vi "configure.vi"(8 "error in (no error)":errorcluster, 11 "SweepDL090926Automation in":refnum<class "SweepDL090926Automation.lvclass">) -> (0 "error out":errorcluster, 3 "SweepDL090926Automation out":refnum<class "SweepDL090926Automation.lvclass">)   [LabVIEW 2010, in "SweepDL090926Automation.lvclass"]
doc: "The dynamic dispatch version of this VI loads and displays the configuration file associated with the plug-in object. The user modify and save the configuration data."
uses:
  SweepDL090926Automation.lvclass
  ImagingMode/GenericImagingMode/GenericImagingMode/GenericImagingMode.lvclass
  SweepDL090926Automation.lvclass/SweepDL090926Automation.ctl
  common/classes/GenericComponent/GenericComponent/GenericComponent.lvclass
panel:
  in  "cancel button":bool
  in  "save button":bool
  in  "edit sequence button":bool
  # "Configure SweepDL090926Automation"
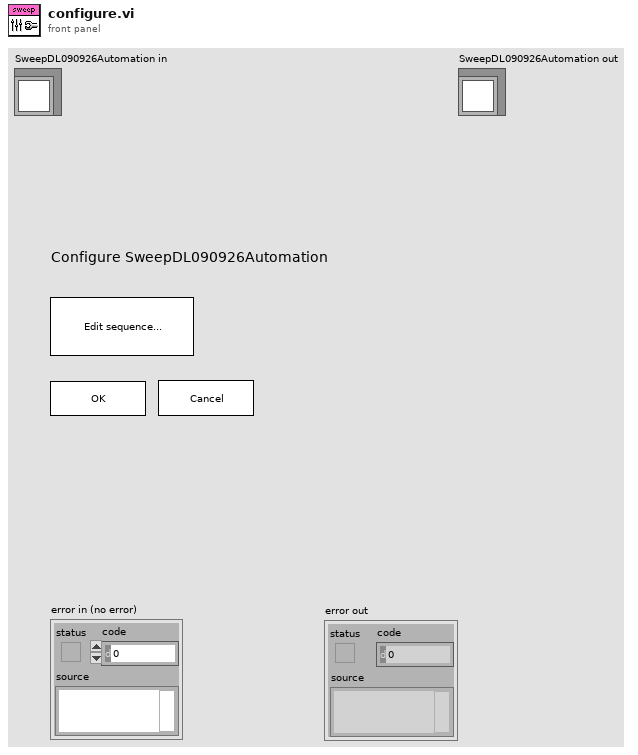
[diagram p1: front panel]
types:
  T1 = typedef "plugin_specification.ctl" = cluster{"class path":string, "configuration":string, "label":string, "settings name":string}
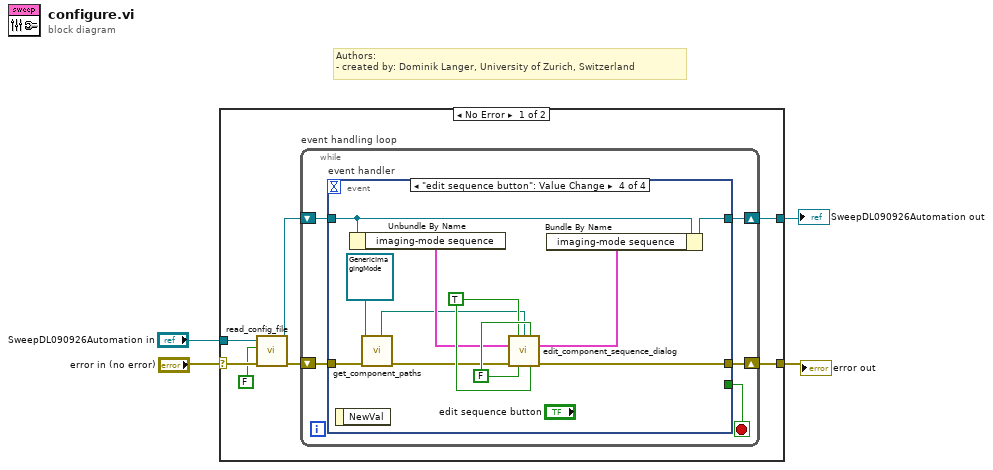
[diagram p0: block diagram]
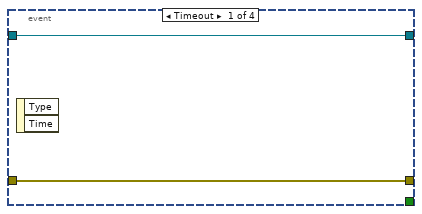
[diagram p2: hidden frame]
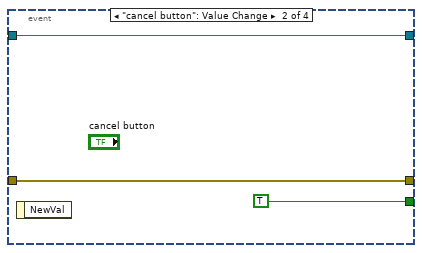
[diagram p3: hidden frame]
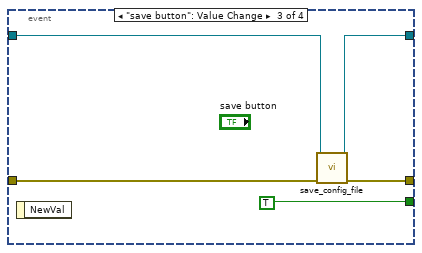
[diagram p4: hidden frame]
diagram:
  # "Authors: \n- created by: Dominik Langer, University of Zurich, Switzerland"
  n1 = case shown="No Error" "error in (no error)" {
    selector: "error in (no error)" -> [w9 w38]
    tunnel: "SweepDL090926Automation in" -> [w6 w39]
    tunnel: [w11 w39] -> w2
    tunnel: [w10 w38] -> w1
    frame No Error {
      n2 = call-dynamic "read_config_file.vi"("error in (no error)"=w9, "force load?"=FALSE, "GenericPlugin in"=w6) -> ("error out"=w8:errorcluster, "GenericPlugin out"=w5:refnum<class "SweepDL090926Automation.lvclass">)  [unwired: 7 in]
      n3 = while "event handling loop" {
        shift-right: [w15] -> w11
        shift-left: w5 -> [w16]
        shift-right: [w13] -> w10
        shift-left: w8 -> [w14]
        stop <- w12 stop-if-true
        n4 = event "event handler" shown="[3] \"edit sequence button\": Value Change" {
          selector: _ -> [_ _ _ _]
          dyn-events: _ -> [_ _ _ _]
          timeout: _ -> [_ _ _ _]
          tunnel: w16 -> [w18 w21 w22 w27]
          tunnel: [w18 w21 w23 w33] -> w15
          tunnel: w14 -> [w17 w20 w25 w31]
          tunnel: [w17 w20 w24 w37] -> w13
          tunnel: [_ TRUE TRUE _] -> w12
          event Timeout {
            n5 = event-data() -> ()  [unwired: 1 in, 2 out]
          }
          event "cancel button": Value Change {
            n6 = event-data() -> ()  [unwired: 1 in, 1 out]
          }
          event "save button": Value Change {
            n7 = event-data() -> ()  [unwired: 1 in, 1 out]
            n8 = call-dynamic "save_config_file.vi"("error in (no error)"=w25, "GenericPlugin in"=w22) -> ("error out"=w24:errorcluster, "GenericPlugin out"=w23:refnum<class "SweepDL090926Automation.lvclass">)  [unwired: 8 in]
          }
          event "edit sequence button": Value Change {
            w35 = TRUE ("show configuration?")
            w36 = FALSE ("choose default?")
            n9 = event-data() -> ()  [unwired: 1 in, 1 out]
            n10 = Unbundle By Name(w27) -> ("imaging-mode sequence"=w34:T1[])
            n11 = call-dynamic "get_component_paths.vi"("error in (no error)"=w31, "GenericComponent in"=refnum<class "GenericImagingMode.lvclass"> refnum ("GenericImagingMode.lvclass")) -> ("error out"=w30:errorcluster, "component type directory"=w29:path)  [unwired: 4 in, 4 out]
            n12 = call "edit_component_sequence_dialog.vi"("show configuration?"=w35, "default folder path"=w29, "show label?"=w36, "component specification list in"=w34, "error in (no error)"=w30, "choose default?"=w36, "show settings?"=w35) -> ("component specification list out"=w32:T1[], "error out"=w37:errorcluster)  [unwired: 6 in, 1 out]
            n13 = Bundle By Name(cluster=w27, "imaging-mode sequence"=w32) -> (w33:refnum<class "SweepDL090926Automation.lvclass">)
          }
        }
      }
    }
    frame Error {
    }
  }
  "error out" <- w1
  "SweepDL090926Automation out" <- w2
